vi "repack-h5.vi"(1 "error in":errorcluster, 2 "dest":path, 3 "source":path) -> (0 "error out":errorcluster)   [LabVIEW 2013]
uses:
  <vilib>/addons/h5labview2/file/H5Fmode.ctl
  <vilib>/addons/h5labview2/file/H5F.lvlib
  <vilib>/addons/h5labview2/attrib/H5A.lvlib
  <vilib>/addons/h5labview2/group/H5G.lvlib
panel:
  # "Repack H5 file"
  # "This VI copies all the contents of an H5 file into another file. This new file will\nbe smaller than the original if it contains \"dead space\"."
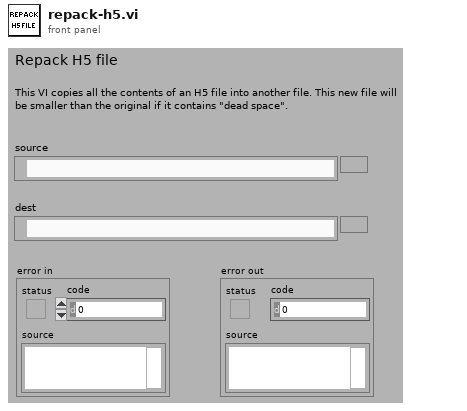
[diagram p1: front panel]
types:
  T1 = typedef "H5F.lvlib/H5Fmode.ctl" = enum16{"read-only", "read-write", "overwrite", "create new", "open or create"}
  T2 = typedef "hid_t.ctl" = i32
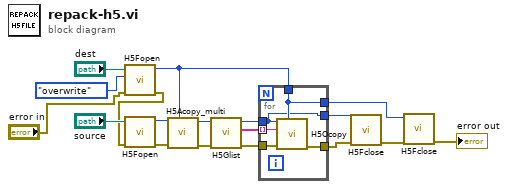
[diagram p0: block diagram]
diagram:
  n1 = call <vilib>:"H5Fopen.vi"("error in (no error)"="error in", "mode (read-only)"=H5Fmode."overwrite", "path"="dest") -> ("error out"=w9:errorcluster, "ref out"=w11:T2)  [unwired: 7 in]
  n2 = call <vilib>:"H5Fopen.vi"("error in (no error)"=w9, "path"="source") -> ("error out"=w8:errorcluster, "ref out"=w12:T2)  [unwired: 8 in]
  n3 = call <vilib>:"H5Acopy_multi.vi"("dest in"=w11, "error in (no error)"=w8, "src in"=w12) -> ("error out"=w7:errorcluster, "src out"=w15:T2)  [unwired: 7 in]
  n4 = call <vilib>:"H5Glist.vi"("error in (no error)"=w7, "ref in"=w15) -> ("error out"=w6:errorcluster, "names"=w13:string[], "ref out"=w14:T2)  [unwired: 6 in, 1 out]
  n5 = for {
    tunnel: w14 -> [w21]
    tunnel: w13 -> [w23] mode=indexing
    tunnel: w11 -> [w22]
    tunnel: [w22] -> w3
    tunnel: [w21] -> w10
    tunnel: w6 -> [w20]
    tunnel: [w19] -> w5
    n6 = call <vilib>:"H5Ocopy.vi"("dest in"=w22, "error in (no error)"=w20, "src name (.)"=w23, "src in"=w21) -> ("error out"=w19:errorcluster)  [unwired: 6 in, 1 out]
  }
  n7 = call <vilib>:"H5Fclose.vi"("error in (no error)"=w5, "ref"=w10) -> ("error out"=w4:errorcluster)  [unwired: 9 in]
  n8 = call <vilib>:"H5Fclose.vi"("error in (no error)"=w4, "ref"=w3) -> ("error out"=→"error out":errorcluster)  [unwired: 9 in]
